vi "mode_sensitivity.vi"(0 "reference":refnum<class "OSA300.lvclass">, 2 "sensitivity":u16=3, 5 "error in (no error)":errorcluster, 7 "ctrl ref":refnum<vi>, 9 "read/write":enum16{"read", "write"}(ring)) -> (14 "duplicate reference":refnum<class "OSA300.lvclass">, 16 "sensitivity out":u16=3, 19 "error out":errorcluster)   [LabVIEW 2010, in "OSA300.lvclass"]
doc: "Sensitivity affect settable gain range, (sensitivity high: gain range = 0-15, and sens low: 0 - 11), and sampling intervall, (nr of samples per reference laser period, sens high: 32, low: 16). Sensitivity high recommended for low power sources or for high performance wavemeter resolution. The update rate, (interferogram read), is lower in high sensitivity mode."
uses:
  OSA300.lvclass
  typeDef/resolution_OSA300.ctl
  OSA.lvclass
  FTSLib.dll
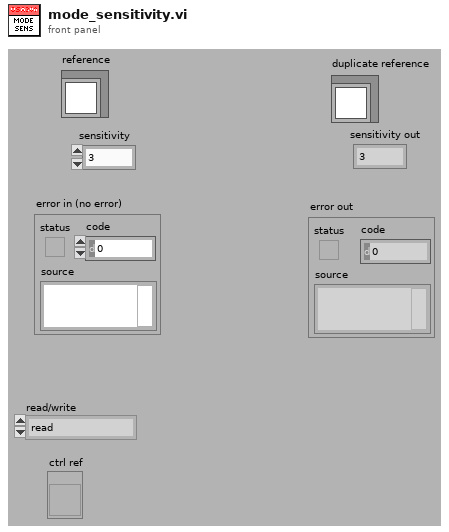
[diagram p1: front panel]
types:
  T1 = typedef "OSA.lvclass/ObjectAttributes.ctl" = cluster{"Stop":bool, "dataType":T2, "spectrometerIdx":u16, "buffer size interferogram":i32, "interferogram":cluster{"new":bool, "plot_x_ min":sgl, "plot_x_max":sgl, "plot_y_min":sgl, "plot_y_max":sgl, "Graph Intrfrgrm":T3, "timeStamp":u32, "signal (%)":dbl, "traces":cluster{"idx":u32, "broadBand":bool, "monoChromatic":bool, "peakToPeakSignal":dbl, "peakToPeakPos":dbl}[], "traces idx last":i32, "contrast (%)":dbl}, "spectrum":cluster{"new":bool, "plot_x_min":sgl, "plot_x_max":sgl, "plot_unit_x":T4, "plot_unit_y":T5, "plot_y_min":sgl, "plot_y_max":sgl, "Graph Spectrum":T3, "timeStamp":u32, "X_VAL_OPTIONS":enum16{"MIN_MAX", "ARRAY"}, "traces":cluster{"idx":u32}[], "traces idx last":i32}, "Thorlabs_OSA_64.lvclass:queue_action.ctlqueue ref":refnum<queue>, "action":T6, "plot zoom step":dbl, "buffer semaphore":T7, "acq stopped":bool, "dataType active":T2, "temperature (degr C)":sgl, "pressure (hPa)":sgl, "rel humidity (%)":sgl, "settings":cluster{"resolution":u16, "sensitivity":u16, "Average":bool, "average nr":u32, "apodisation":T8, "acq delay (ms)":u32, "airMesure":T9, "wmtr on":bool, "intfgrm_smooth_width":u16, "intfgrm_smooth_nrOfPasses":u16, "intfgrm_smooth":T10, "phaseCorrection":T11, "zeroFill":u8, "spectr_smooth":T10, "spectr_smooth_width":u16, "spectr_smooth_nrOfPasses":u16, "resolution (/cm)":sgl, "REF wavelength, (nm)":dbl, "gain_idx":u16, "gainAuto":bool, "gain_relative":dbl, "PD sensitivity mode":T12, "PD senseMode implemented":bool, "SensorTemperature implemented":bool, "SensorPressure implemented":bool, "SensorHumidity implemented":bool, "attenuationAuto":bool, "attenuationOnOff":bool, "attenuationAvailable":bool, "offsetAvailable":bool, "offset":i32, "offset max":u16, "contrastAvailable":bool}, "peaks position":sgl[], "peaks width":sgl[], "peaks height":sgl[], "peaks max nr":u32, "peaks latest nr":i32, "peaks new":bool, "power":dbl, "power new":bool, "path":string, "wavelength (WNr)":dbl, "wavelength new":bool, "buffer size spectrum":i32, "status":string, "vi reference":refnum<vi>, "funcPointer":u64, "libraryPointer":u64, "singleAcquisition":bool, "coherenceLength (cm)":dbl, "coherenceLength new":bool, "spectrometer model":string, "spectrometer serial nr":string, "peaks thld left":sgl[], "peaks thld right":sgl[], "coherenceLength error (cm)":dbl, "ADC bits":u16, "peaks position centroid":sgl[], "peaks height centroid":sgl[], "OSA series":T13, "channel index spectrum":u16, "spectrometer rangeLow, (/cm)":dbl, "spectrometer rangeHigh, (/cm)":dbl, "channel index interferogram":u16, "virtualSource":bool, "sweep restart":bool}
  T2 = typedef "OSA.lvclass/acq_dataType.ctl" = enum16{"none", "interferogram", "spectrum"}
  T3 = typedef "OSA.lvclass/graph_intensity.ctl" = refnum<vi>
  T4 = typedef "OSA.lvclass/spectrum_x_unit.ctl" = enum16{"wavenr/cm", "THz", "eV", "nm_air", "nm_vac"}
  T5 = typedef "OSA.lvclass/y_unit.ctl" = enum16{"ADC counts", "dBm pwr absolute", "dBm pwr density", "mW pwr absolute", "mW pwr density"}
  T6 = typedef "OSA.lvclass/queue_action.ctl" = enum16{"none", "stop", "GUI_plotInterferogram", "GUI_plotSpectrum", "GUI_plotInterferogramRescale", "GUI_plotSpectrumRescale", "GUI_plotInterferogramReset", "GUI_plotSpectrumReset", "GUI_plotInterferogramAutoScaleY", "GUI_plotSpectrumAutoScaleY", "GUI_plotInterferogramZoomOut", "GUI_plotSpectrumZoomOut", "GUI_plotInterferogramPane", "GUI_plotSpectrumPane", "GUI_plotInterferogramZoomMouse", "GUI_plotSpectrumZoomMouse", "GUI_plotSpectrumFSRY", "GUI_plotInterferogramFSRY", "GUI_spectrumChannelType", "GUI_channel", "ENVIRONMENT temperature", "ENVIRONMENT pressure", "MODE_resolution set", "MODE_resolution get", "MODE_sensitivity set", "MODE_sensitivity get", "MODE_PDTemperature set", "MODE_PDTemperature get", "REBOOT/RESET firmware", "ACQASYNC_acquireSingleSpectrum", "ACQASYNC_continuous start", "ACQASYNC_continuous stop\n", "ACQASYNC_get last interferogram", "ACQASYNC_get last spectrum", "ACQASYNC_get last waveNr", "ACQOPT_interferogram smoothing set", "ACQOPT_interferogram smoothing get", "ACQOPT_spectrum smoothing set", "ACQOPT_spectrum smoothing get", "ACQOPT_apodisation type set", "ACQOPT_apodisation type get", "ACQOPT_phase correction type set", "ACQOPT_phase correction type get", "ACQOPT_acqIntervall_set", "ACQOPT_acqIntervall_get", "ACQOPT_average spectrum set", "ACQOPT_average spectrum get", "ACQOPT_rolling average set", "ACQOPT_rolling average get", "ACQOPT_zero fill factor set", "ACQOPT_zero fill factor get", "ACQOPT_cycle counting set", "ACQOPT_cycle counting get", "ACQOPT_air measure option set", "ACQOPT_air measure option get", "ACQOPT_gainLevel auto get", "ACQOPT_gainLevel auto set", "ACQOPT_gainLevel get", "ACQOPT_gainLevel set", "ACQOPT_offset set", "ACQOPT_attenuator_auto_set", "ACQOPT_attenuator_set", "ACQOPT_getAll", "INSTRUMENT_PROPERTY_range_WaveNr_min", "INSTRUMENT_PROPERTY_range_WaveNr_max", "INSTRUMENT_PROPERTY_reference_wavelength_cm^-1", "INSTRUMENT_PROPERTY_samplesPerRefPeriod", "INSTRUMENT_PROPERTY_resolution_waveNrPercm", "INSTRUMENT_PROPERTY_availableGainLevels", "INSTRUMENT_PROPERTY_status", "CONVERT", "ANALYSE_POWER", "ANALYSE_PEAKS", "ANALYSE_WAVELENGTH", "ANALYSE_SPECTRUM", "ANALYSE_INTERFEROGRAM", "ANALYSE_COHERENCE_LENGTH", "MATH", "MATH_power", "MATH_peaks", "FILE", "miscellaneous"}
  T7 = typedef "Semaphore RefNum" = refnum<k1>
  T8 = typedef "OSA.lvclass/apodisation.ctl" = enum16{"NONE", "NORTON_BEER_WEAK", "NORTON_BEER_MEDIUM", "NORTON_BEER_STRONG", "TRIANGULAR", "COSINE", "HANN", "HAMMING", "BLACKMANHARRIS3", "BLACKMANHARRIS4", "GAUSSIAN"}
  T9 = typedef "OSA.lvclass/airMeasure.ctl" = enum16{"TEMPERATURE", "PRESSURE"}
  T10 = typedef "OSA20X_misc.lvlib/interferogram_smoothing.ctl" = enum16{"NONE", "BINOMIAL", "SAVITSKY_GOLAY", "FOURIER", "MOVING_AVERAGE", "GAUSSIAN"}
  T11 = typedef "OSA.lvclass/phaseCorrection.ctl" = enum16{"NONE", "MERTZ", "FORMAN", "MERTZ_FILE", "FORMAN_FILE", "FUTURE COMP."}
  T12 = typedef "OSA20X_misc.lvlib/PDTemperatureMode.ctl" = enum16{"cool: better sensitivity/noise floor", "warm: extended wl range"}
  T13 = typedef "OSA.lvclass/OSA_series.ctl" = enum16{"OSA200", "OSA300", "UNKNOWN"}
  T14 = typedef "OSA300.lvclass/resolution_OSA300.ctl" = enum16{"low", "medium low", "medium high", "high"}
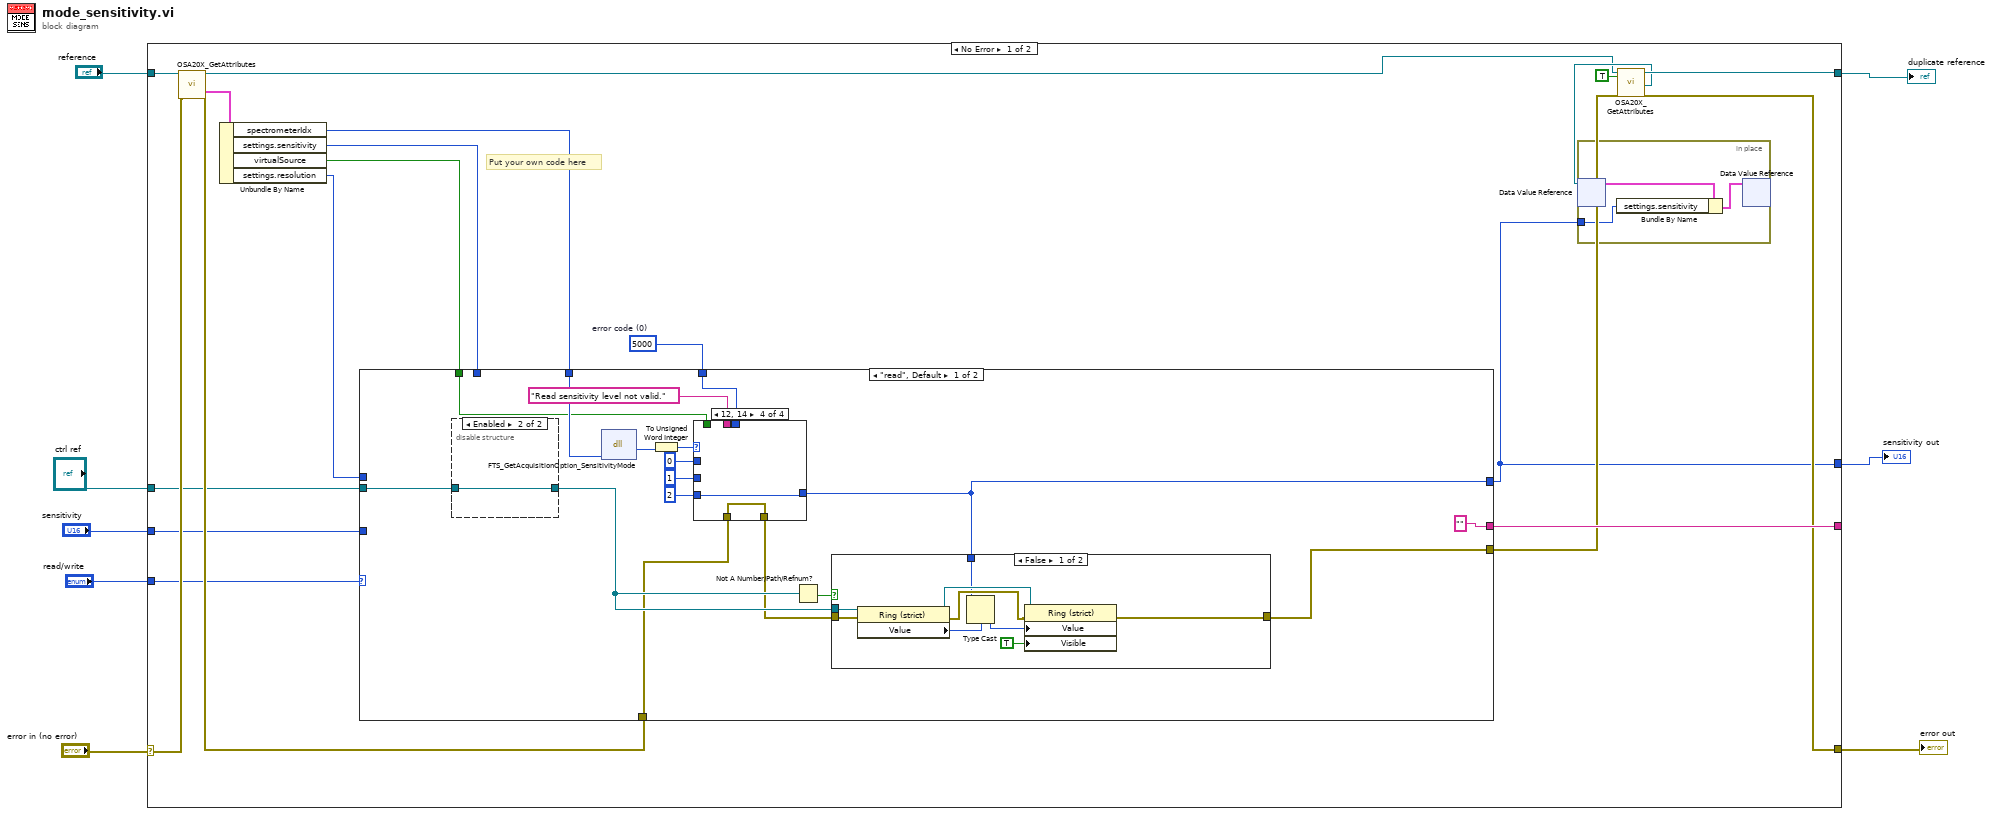
[diagram p0: block diagram]
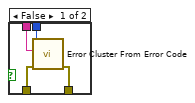
[diagram p3: hidden frame]
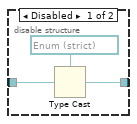
[diagram p6: hidden frame]
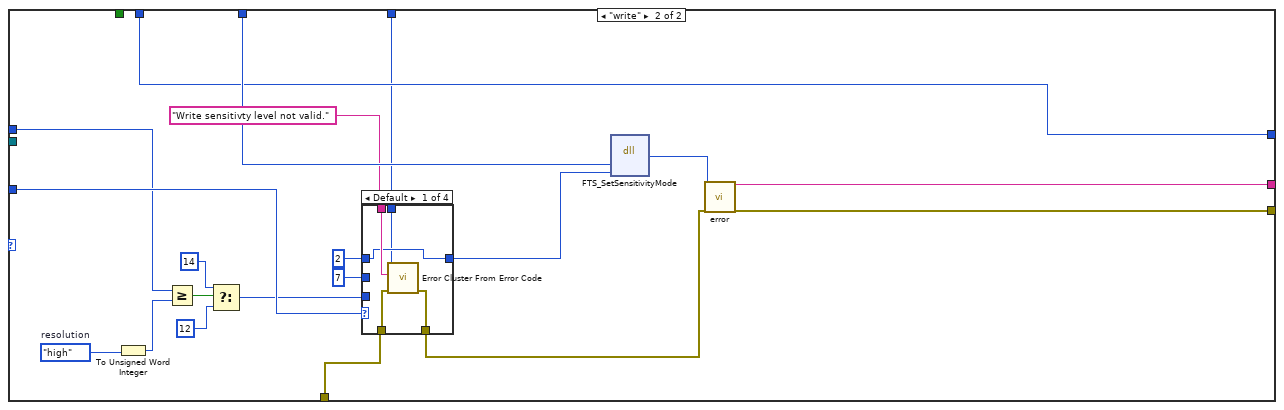
[diagram p8: hidden frame]
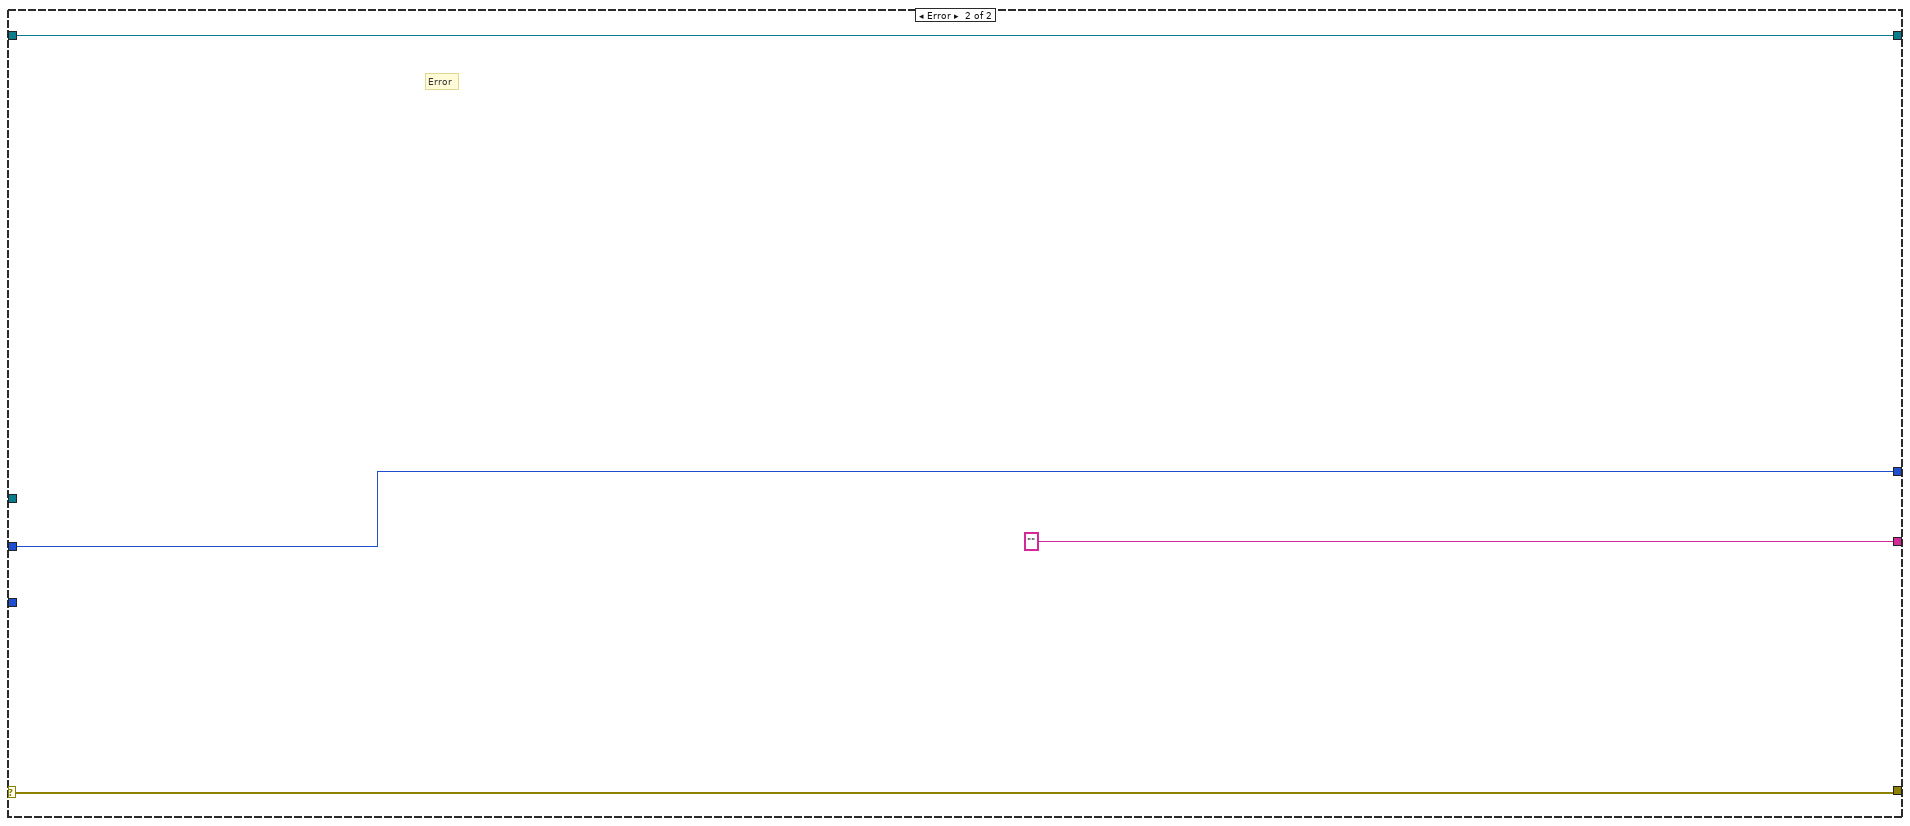
[diagram p12: hidden frame]
diagram:
  n1 = case shown="No Error" "error in (no error)" {
    selector: "error in (no error)" -> [w27 w113]
    tunnel: [w19 w113] -> w1
    tunnel: "reference" -> [w28 w114]
    tunnel: [w21 w114] -> w3
    tunnel: "sensitivity" -> [w22 w111]
    tunnel: [w25 "" ("status")] -> _
    tunnel: "read/write" -> [w23 _]
    tunnel: [w14 w111] -> w2
    tunnel: "ctrl ref" -> [w12 _]
    frame No Error {
      w11 = 5000  # error code (0)
      # "Put your own code here"
      n2 = call "OSA20X_GetAttributes.vi"("reference in"=w28, "error in (no error)"=w27) -> ("reference out"=w13:refnum<class "OSA300.lvclass">, "Data"=w16:T1, "error out"=w26:errorcluster)  [unwired: 14 in, 1 out]
      n3 = Unbundle By Name(w16) -> ("spectrometerIdx"=w24:u16, "settings.sensitivity"=w18:u16, "virtualSource"=w10:bool, "settings.resolution"=w9:u16)
      n4 = case shown="\"read\", Default" w23 {
        tunnel: w26 -> [w36 w90]
        tunnel: [w45 w96] -> w20
        tunnel: w22 -> [_ w94]
        tunnel: ["" ("status") w98] -> w25
        tunnel: w24 -> [w44 w97]
        tunnel: [w37 w95] -> w14
        tunnel: w18 -> [_ w95]
        tunnel: w12 -> [w42 _]
        tunnel: w11 -> [w33 w87]
        tunnel: w10 -> [w32 _]
        tunnel: w9 -> [_ w86]
        frame "read", Default {
          n5 = disable-structure shown="Enabled" {
            disable-tunnel: [w68 w69] -> w46
            disable-tunnel: w42 -> [w66 w69]
            frame Disabled {
              n6 = Type Cast(type=refnum<vi> refnum ("sensitivity 2"), x=w66) -> (*(type *) &x=w68:refnum<vi>)
            }
            frame Enabled {
            }
          }
          n7 = dll-call lib="FTSLib.dll" fn="FTS_GetAcquisitionOption_SensitivityMode"("spectrIdx"=w44) -> ("return type"=w43:i32)  [unwired: 4 in, 2 out]
          n8 = To Unsigned Word Integer(number=w43) -> (unsigned 16bit integer=w41:u16)
          n9 = case shown="12, 14" w41 {
            tunnel: u16 0 ("sensitivityMode") -> [w51 w61 _ _]
            tunnel: u16 1 ("sensitivityMode") -> [_ _ w63 _]
            tunnel: [w51 w61 w63 w65] -> w37
            tunnel: u16 2 ("sensitivityMode") -> [_ _ _ w65]
            tunnel: w36 -> [w54 w60 w62 w64]
            tunnel: [w53 w60 w62 w64] -> w35
            tunnel: "Read sensitivity level not valid." ("error message (\"\")") -> [w52 _ _ _]
            tunnel: w33 -> [w50 _ _ _]
            tunnel: w32 -> [w49 _ _ _]
            frame Default {
              n10 = case shown="True" w49 {
                tunnel: w54 -> [w58 w59]
                tunnel: [w57 w59] -> w53
                tunnel: w52 -> [w56 _]
                tunnel: w50 -> [w55 _]
                frame False {
                  n11 = call <vilib>:"Error Cluster From Error Code.vi"("error in (no error)"=w58, "error message (\"\")"=w56, "error code (0)"=w55) -> ("error out"=w57:errorcluster)  [unwired: 6 in]
                }
                frame True {
                }
              }
            }
            frame 2 {
            }
            frame 7 {
            }
            frame 12, 14 {
            }
          }
          n12 = Not A Number/Path/Refnum?(number/path/refnum=w46) -> (NaN/Path/Refnum?=w47:bool)
          n13 = case shown="False" w47 {
            tunnel: w35 -> [w78 w79]
            tunnel: w46 -> [w77 _]
            tunnel: [w72 w79] -> w45
            tunnel: w37 -> [w70 _]
            frame False {
              n14 = property class="Ring (strict)"(reference=w77, error in=w78) -> (reference out=w71:refnum<vi>, error out=w73:errorcluster, "Value"=w76:u16)
              n15 = Type Cast(type=w76, x=w70) -> (*(type *) &x=w75:u16)
              n16 = property class="Ring (strict)"(reference=w71, error in=w73, "Value"=w75, "Visible"=TRUE) -> (error out=w72:errorcluster)  [unwired: 1 out]
            }
            frame True {
            }
          }
        }
        frame "write" {
          w80 = resolution_OSA300."high"  # resolution
          n17 = To Unsigned Word Integer(number=w80) -> (unsigned 16bit integer=w85:u16)
          n18 = Greater Or Equal?(x=w86, y=w85) -> (x >= y?=w84:bool)
          n19 = Select(t=u16 14 ("sensitivityMode"), s=w84, f=u16 12 ("sensitivityMode")) -> (s? t:f=w82:u16)
          n20 = case shown="Default" w94 {
            tunnel: u16 2 ("sensitivityMode") -> [w101 w106 _ _]
            tunnel: [w101 w106 w108 w110] -> w93
            tunnel: u16 7 ("sensitivityMode") -> [_ _ w108 _]
            tunnel: w82 -> [_ _ _ w110]
            tunnel: w90 -> [w104 w105 w107 w109]
            tunnel: [w103 w105 w107 w109] -> w89
            tunnel: "Write sensitivty level not valid." ("error message (\"\")") -> [w102 _ _ _]
            tunnel: w87 -> [w100 _ _ _]
            frame Default {
              n21 = call <vilib>:"Error Cluster From Error Code.vi"("error in (no error)"=w104, "error message (\"\")"=w102, "error code (0)"=w100) -> ("error out"=w103:errorcluster)  [unwired: 6 in]
            }
            frame 0 {
            }
            frame 1 {
            }
            frame 2 {
            }
          }
          n22 = dll-call lib="FTSLib.dll" fn="FTS_SetSensitivityMode"("spectrIdx"=w97, "sensitivityMode"=w93) -> ("return type"=w99:i32)  [unwired: 5 in, 2 out]
          n23 = call "error.vi"("result code"=w99, "error in (no error)"=w89) -> ("status"=w98:string, "error out"=w96:errorcluster)  [unwired: 15 in, 1 out]
        }
      }
      n24 = call "OSA20X_GetAttributes.vi"("reference in"=w13, "OnlyGetDvrReference(False)"=TRUE, "error in (no error)"=w20) -> ("reference out"=w21:refnum<class "OSA300.lvclass">, "DataRef"=w15:refnum<data-value>, "error out"=w19:errorcluster)  [unwired: 13 in, 1 out]
      n25 = in-place {
        in-place-border: w14 -> [w30]
        n26 = in-place-dvr #1(w15) -> (w31:T1)  [unwired: 1 out]
        n27 = Bundle By Name(cluster=w31, "settings.sensitivity"=w30) -> (w29:T1)
        n28 = in-place-dvr #1(w29) -> ()  [unwired: 2 out]
      }
    }
    frame Error {
      # "Error"
    }
  }
  "error out" <- w1
  "duplicate reference" <- w3
  "sensitivity out" <- w2
